vi "Benchmark SV Send  LV2012 - NI Verified - 10 Byte.vi"() -> ()   [LabVIEW 2015]
panel:
  out "10 byte":u64[](array[numeric])
  in  "Reset":bool
  out "Tries":u32
  out "Average Delay (ms)":dbl
  out "Delay (ms)":u32
  in  "stop":bool
  # "Overview:  Coding that exemplifies how to benchmark the communication of Shared Variables.\nRequirements: LabVIEW 2012 or compatible\nInstructions:\n1.  Run the \"Benchmark SV Receive LV2012 - NI Verified.vi\"\n2. Run this VI\n3. Watch the amount of time it takes to communicate\n4. Stop both VIs"
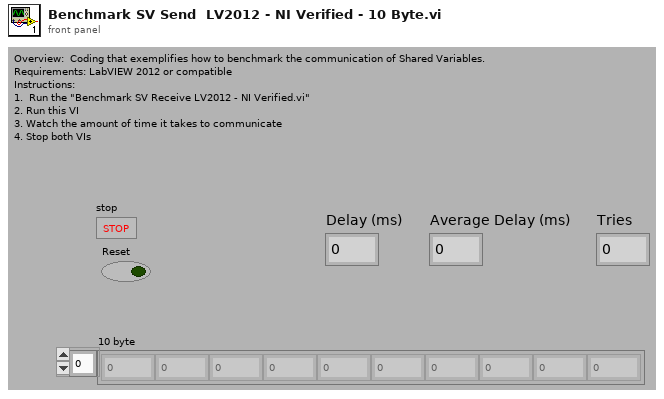
[diagram p1: front panel]
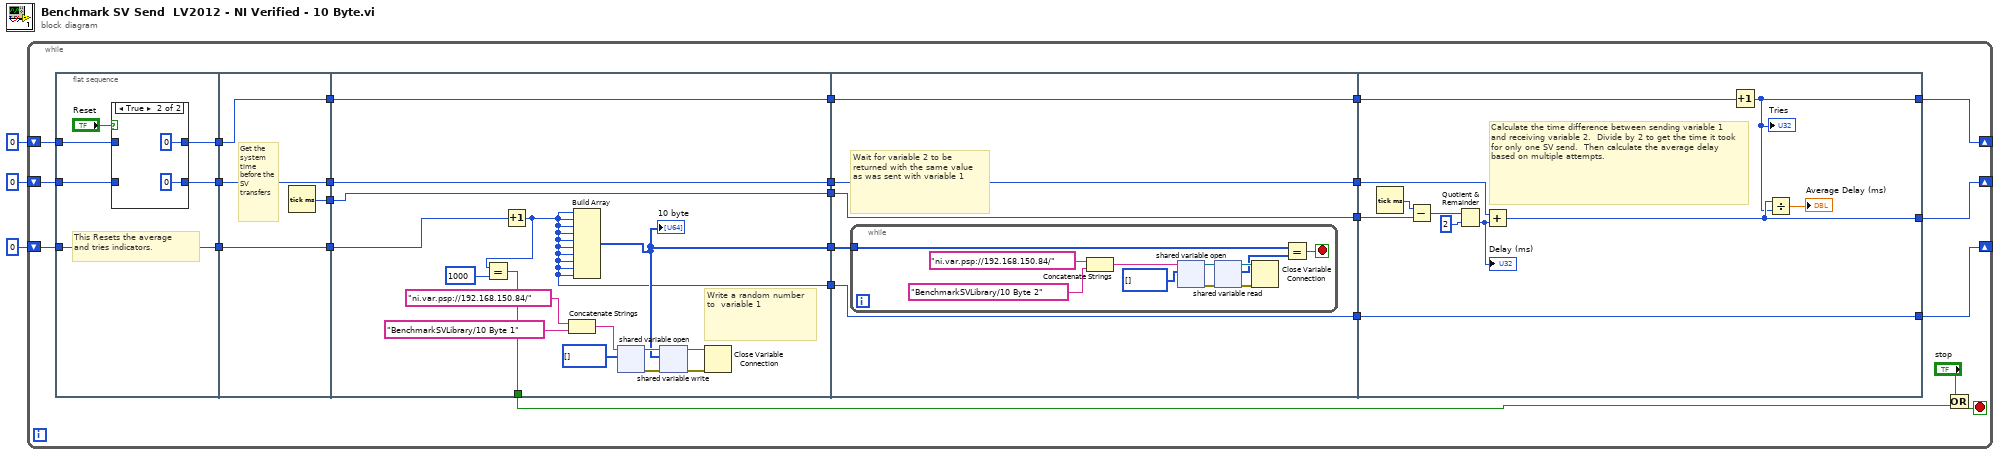
[diagram p0: block diagram]
diagram:
  n1 = while {
    shift-right: [w25] -> _
    shift-left: u32 0 -> [w13]
    shift-right: [w22] -> _
    shift-left: u32 0 -> [w14]
    shift-right: [w7] -> _
    shift-left: u64 0 -> [w10]
    stop <- w6 stop-if-true
    n2 = flat-sequence {
      tunnel: w13 -> [w34]
      tunnel: [w33] -> w18
      tunnel: [w31] -> w16
      tunnel: w14 -> [w30]
      tunnel: [w29] -> w11
      tunnel: w10 -> [w29]
      tunnel: [w40] -> w19
      tunnel: w18 -> [w42]
      tunnel: [w42] -> w17
      tunnel: w16 -> [w41]
      tunnel: [w41] -> w15
      tunnel: [w39] -> w12
      tunnel: w11 -> [w39]
      tunnel: [w44] -> w28
      tunnel: [w58] -> w27
      tunnel: [w57] -> w23
      tunnel: [w56] -> w20
      tunnel: w19 -> [w58]
      tunnel: w17 -> [w57]
      tunnel: w15 -> [w56]
      tunnel: w12 -> [w48]
      tunnel: [w43] -> w8
      tunnel: [w45] -> w4
      tunnel: w28 -> [w63]
      tunnel: [w62] -> w26
      tunnel: w27 -> [w62]
      tunnel: [w61] -> w24
      tunnel: w23 -> [w61]
      tunnel: [w60] -> w21
      tunnel: w20 -> [w60]
      tunnel: [w59] -> w9
      tunnel: w8 -> [w59]
      tunnel: w26 -> [w84]
      tunnel: [w77] -> w25
      tunnel: w24 -> [w79]
      tunnel: [w76] -> w22
      tunnel: w21 -> [w83]
      tunnel: w9 -> [w75]
      tunnel: [w75] -> w7
      frame #0 {
        # "This Resets the average \nand tries indicators."
        n3 = case shown="True" "Reset" {
          tunnel: [w36 u32 0] -> w33
          tunnel: w34 -> [w36 _]
          tunnel: [w35 u32 0] -> w31
          tunnel: w30 -> [w35 _]
          frame False {
          }
          frame True {
          }
        }
      }
      frame #1 {
        # "Get the system time before the SV transfers"
        n4 = Tick Count (ms)() -> (millisecond timer value=w40:u32)
      }
      frame #2 {
        # "Write a random number to  variable 1"
        n5 = Increment(x=w48) -> (x+1=w43:u64)
        n6 = Equal?(x=w43, y=u64 1000) -> (x = y?=w45:bool)
        n7 = Concatenate Strings("ni.var.psp://192.168.150.84/" ("string"), "BenchmarkSVLibrary/10 Byte 1") -> (w51:string)
        n8 = Build Array(w43, w43, w43, w43, w43, w43, w43, w43, w43, w43) -> (w44:u64[])
        "10 byte" <- w44
        n9 = shared-variable-open(w51, u64[] [] ("appended array")) -> (w55:refnum<k21>, w52:errorcluster)  [unwired: 2 in]
        n10 = shared-variable-write(w55, w52, w44) -> (w53:refnum<k21>, w54:errorcluster)
        n11 = Close Variable Connection(8:w54, 11:w53) -> ()  [unwired: 1 out]
      }
      frame #3 {
        # "Wait for variable 2 to be returned with the same value as was sent with variable 1"
        n12 = while {
          tunnel: w63 -> [w65]
          stop <- w74 stop-if-true
          n13 = Concatenate Strings("ni.var.psp://192.168.150.84/" ("string"), "BenchmarkSVLibrary/10 Byte 2") -> (w72:string)
          n14 = shared-variable-open(w72, u64[] [] ("appended array")) -> (w68:refnum<k21>, w71:errorcluster)  [unwired: 2 in]
          n15 = shared-variable-read(w68, w71) -> (w70:refnum<k21>, w69:errorcluster, w67:u64[])  [unwired: 1 out]
          n16 = Close Variable Connection(8:w69, 11:w70) -> ()  [unwired: 1 out]
          n17 = Equal?(x=w65, y=w67) -> (x = y?=w74:bool)
        }
      }
      frame #4 {
        # "Calculate the time difference between sending variable 1 and receiving variable 2.  Divide by 2 to get the time it took for only one SV send.  Then calculate the average delay based on multiple attempts."
        n18 = Tick Count (ms)() -> (millisecond timer value=w85:u32)
        n19 = Subtract(x=w85, y=w84) -> (x-y=w82:u32)
        n20 = Quotient & Remainder(x=w82, y=u32 2) -> (floor(x/y)=w80:u32)  [unwired: 1 out]
        "Delay (ms)" <- w80
        n21 = Add(x=w79, y=w80) -> (x+y=w77:u32)
        n22 = Increment(x=w83) -> (x+1=w76:u32)
        "Tries" <- w76
        n23 = Divide(x=w77, y=w76) -> (x/y=→"Average Delay (ms)":dbl)
      }
    }
    n24 = Or(x="stop", y=w4) -> (x .or. y?=w6:bool)
  }
